vi "Mouse Move Event_demo.vi"() -> ()   [LabVIEW 2012]
panel:
  out "error out":errorcluster
  in  "error in":errorcluster
  in  "Position":cluster{"dx":u32, "dy":u32}
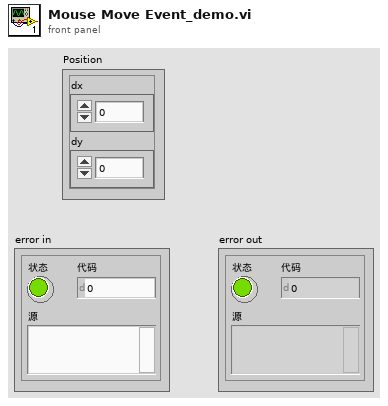
[diagram p1: front panel]
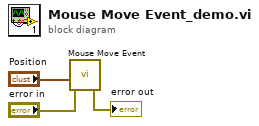
[diagram p0: block diagram]
diagram:
  n1 = call "Mouse Move Event.vi"("error in"="error in", "Position"="Position") -> ("error out"=→"error out":errorcluster)  [unwired: 9 in]
